vi "Display Dialog.vi"(8 "error in (no error)":errorcluster, 9 "Data":variant, 10 "Argument":string, 11 "State Data":T1) -> (0 "error out":errorcluster, 1 "States at Back":string, 2 "States at Front":string, 3 "State Data out":T1)   [LabVIEW 2020, in "MacroAssert.lvlib"]
doc: "Updates one or more elements of <B>State Data</B> based on <B>Argument</B> and <B>Data</B>."
uses:
  MacroAssert.lvlib
  Classes/Macro/Macro.lvclass
  Custom Errors/Custom Errors.lvlib
  CTLs/Edit Action.ctl
  <vilib>/Utility/miscctls.llb/LVRowAndColumnUnsignedTypeDef.ctl
  <vilib>/Platform/browser.llb/Open URL in Default Browser (string).vi
  CTLs/FGV Actions.ctl
  CTLs/Refs.ctl
  CTLs/Report Data.ctl
  CTLs/Config.ctl
  CTLs/State Data.ctl
  CTLs/App Instance.ctl
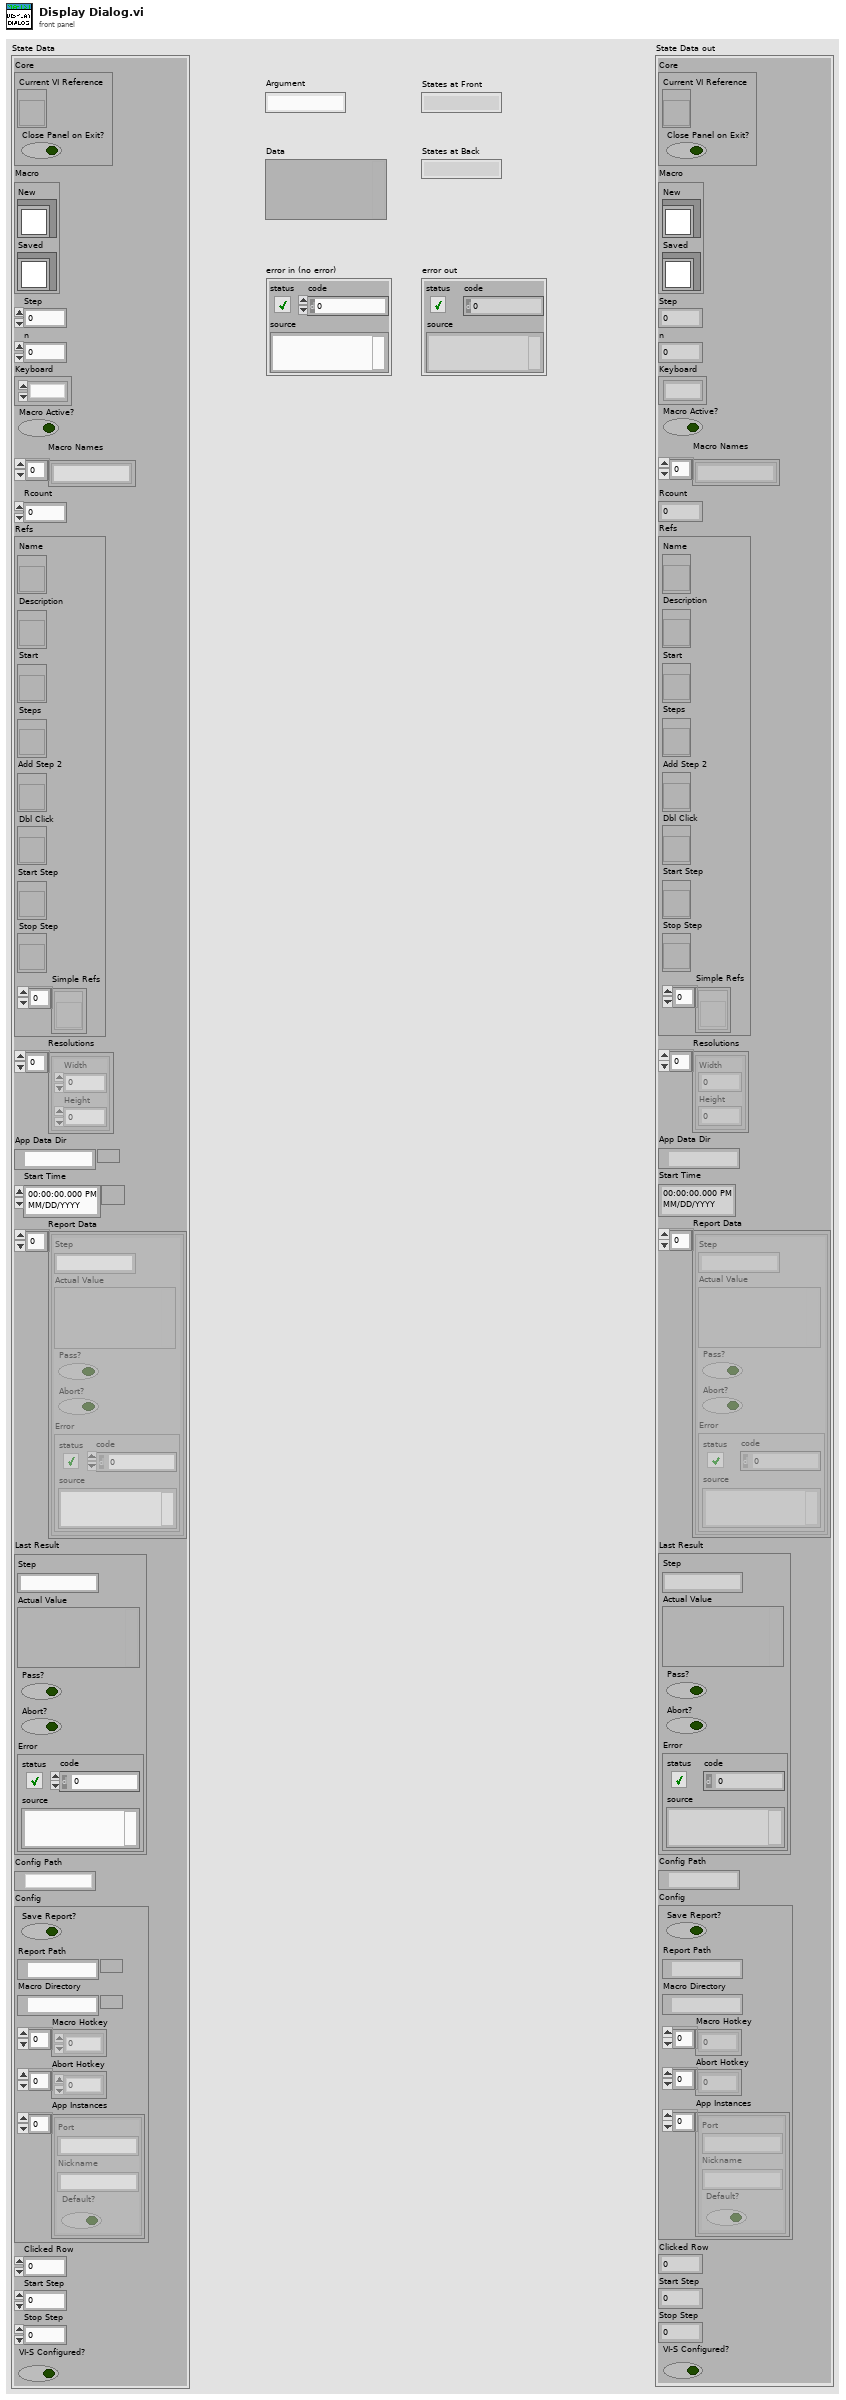
[diagram p1: front panel]
types:
  T1 = typedef "MacroAssert.lvlib/State Data.ctl" = cluster{"Core":cluster{"Current VI Reference":refnum<vi>, "Close Panel on Exit?":bool}, "Macro":cluster{"New":refnum<class "Macro.lvclass">, "Saved":refnum<class "Macro.lvclass">}, "Step":i32, "n":i32, "Keyboard":refnum<k1>, "Macro Active?":bool, "Macro Names":string[], "Rcount":i32, "Refs":T2, "Resolutions":cluster{"Width":i16, "Height":i16}[], "App Data Dir":path, "Start Time":timestamp, "Report Data":T3[], "Last Result":T3, "Config Path":path, "Config":T4, "Clicked Row":i32, "Start Step":i32, "Stop Step":i32, "VI-S Configured?":bool}
  T2 = typedef "MacroAssert.lvlib/Refs.ctl" = cluster{"Name":refnum<vi>, "Description":refnum<vi>, "Start":refnum<vi>, "Steps":refnum<vi>, "Add Step 2":refnum<vi>, "Dbl Click":refnum<vi>, "Start Step":refnum<vi>, "Stop Step":refnum<vi>, "Simple Refs":refnum<vi>[]}
  T3 = typedef "MacroAssert.lvlib/Report Data.ctl" = cluster{"Step":string, "Actual Value":variant, "Pass?":bool, "Abort?":bool, "Error":errorcluster}
  T4 = typedef "MacroAssert.lvlib/Config.ctl" = cluster{"Save Report?":bool, "Report Path":path, "Macro Directory":path, "Macro Hotkey":enum16{"0", "1", "2", "3", "4", "5", "6", "7", "8", "9", "A", "B", "C", "D", "E", "F", "G", "H", "I", "J", "K", "L", "M", "N", "O", "P", "Q", "R", "S", "T", "U", "V", "W", "X", "Y", "Z", "F1", "F2", "F3", "F4", "F5", "F6", "F7", "F8", "F9", "F10", "F11", "F12", "F13", "F14", "F15", "ADD", "BACK", "BACKSLASH", "CAPITAL", "COMMA", "DECIMAL", "DELETE", "DIVIDE", "DOWN", "END", "EQUALS", "ESCAPE", "GRAVE (`)", "HOME", "INSERT", "LBRACKET", "LCONTROL", "LEFT", "L ALT", "LSHIFT", "LWIN", "MINUS", "MULTIPLY", "NEXT", "NUMLOCK", "NUMPAD_0", "NUMPAD_1", "NUMPAD_2", "NUMPAD_3", "NUMPAD_4", "NUMPAD_5", "NUMPAD_6", "NUMPAD_7", "NUMPAD_8", "NUMPAD_9", "PAUSE", "PERIOD", "PRIOR (PG UP)", "RBRACKET", "RCONTROL", "RETURN", "RIGHT", "R ALT", "RSHIFT", "RWIN", "SCROLL", "SEMICOLON", "SLASH", "SPACE", "SUBTRACT", "TAB", "UP", "ENTER (num pad)", "' (quote)"}[], "Abort Hotkey":enum16{"0", "1", "2", "3", "4", "5", "6", "7", "8", "9", "A", "B", "C", "D", "E", "F", "G", "H", "I", "J", "K", "L", "M", "N", "O", "P", "Q", "R", "S", "T", "U", "V", "W", "X", "Y", "Z", "F1", "F2", "F3", "F4", "F5", "F6", "F7", "F8", "F9", "F10", "F11", "F12", "F13", "F14", "F15", "ADD", "BACK", "BACKSLASH", "CAPITAL", "COMMA", "DECIMAL", "DELETE", "DIVIDE", "DOWN", "END", "EQUALS", "ESCAPE", "GRAVE (`)", "HOME", "INSERT", "LBRACKET", "LCONTROL", "LEFT", "L ALT", "LSHIFT", "LWIN", "MINUS", "MULTIPLY", "NEXT", "NUMLOCK", "NUMPAD_0", "NUMPAD_1", "NUMPAD_2", "NUMPAD_3", "NUMPAD_4", "NUMPAD_5", "NUMPAD_6", "NUMPAD_7", "NUMPAD_8", "NUMPAD_9", "PAUSE", "PERIOD", "PRIOR (PG UP)", "RBRACKET", "RCONTROL", "RETURN", "RIGHT", "R ALT", "RSHIFT", "RWIN", "SCROLL", "SEMICOLON", "SLASH", "SPACE", "SUBTRACT", "TAB", "UP", "ENTER (num pad)", "' (quote)"}[], "App Instances":T5[]}
  T5 = typedef "MacroAssert.lvlib/App Instance.ctl" = cluster{"Port":string, "Nickname":string, "Default?":bool}
  T6 = typedef "MacroAssert.lvlib/FGV Actions.ctl" = enum16{"Read", "Write"}
  T7 = typedef "MacroAssert.lvlib/Edit Action.ctl" = enum16{"Add", "Insert", "Modify", "Delete", "Insert Before", "Insert After", "Modify 2", "Delete 2", "Clear All"}
  T8 = typedef "LVRowAndColumnUnsignedTypeDef.ctl" = cluster{"Row":u32, "Column":u32}
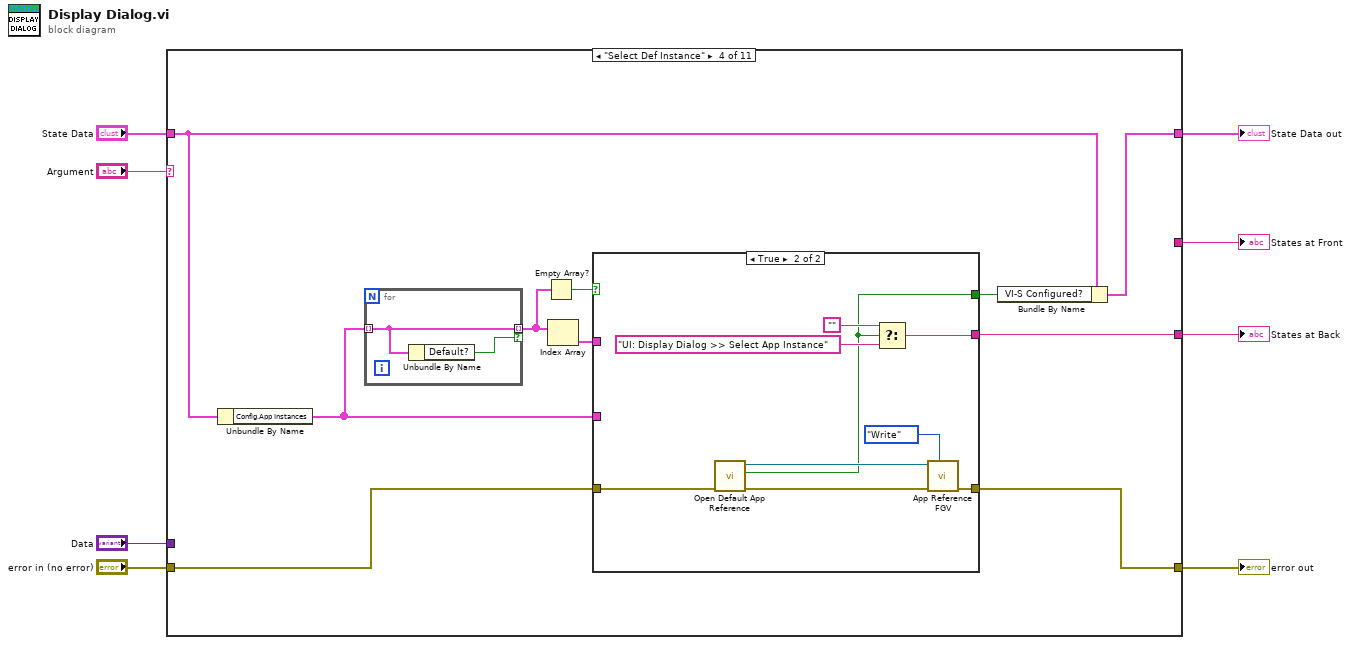
[diagram p0: block diagram]
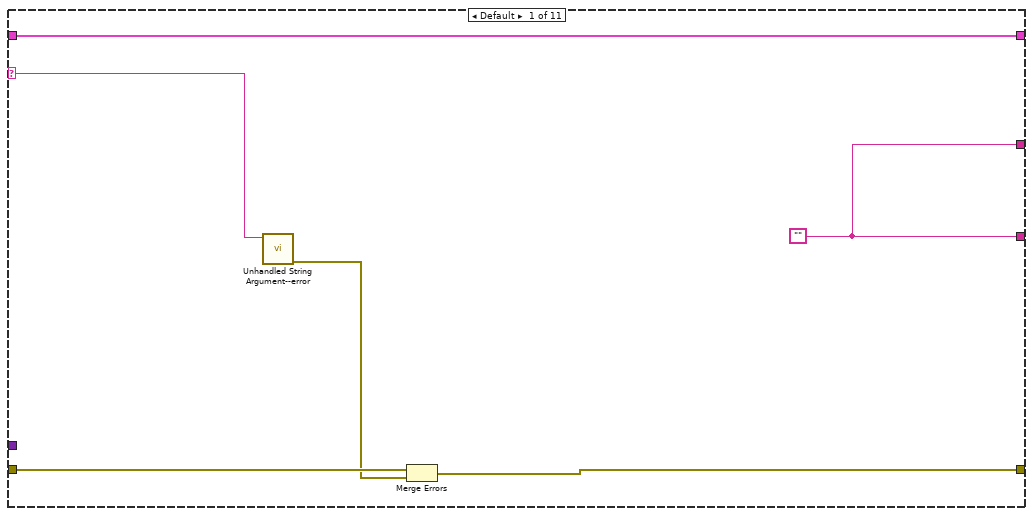
[diagram p2: hidden frame]
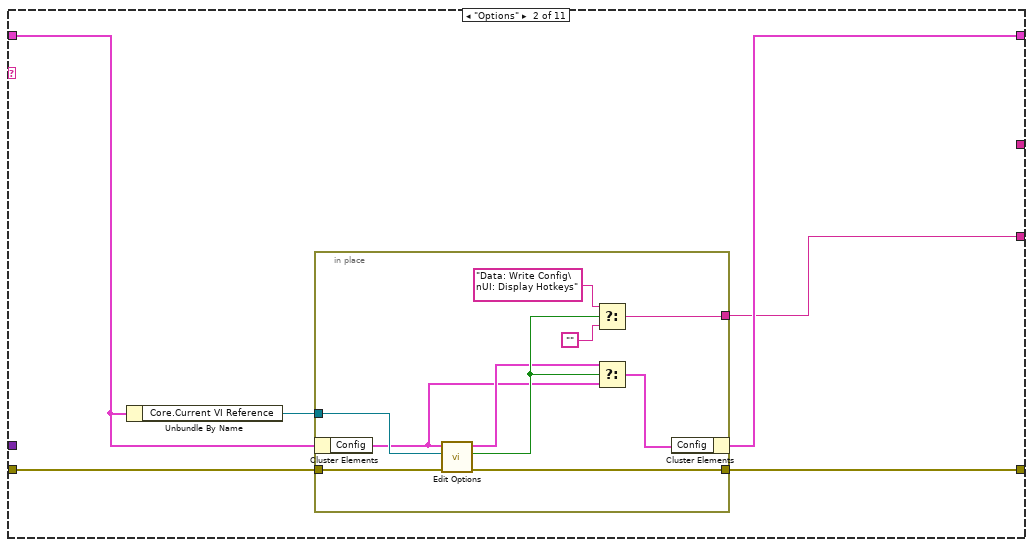
[diagram p3: hidden frame]
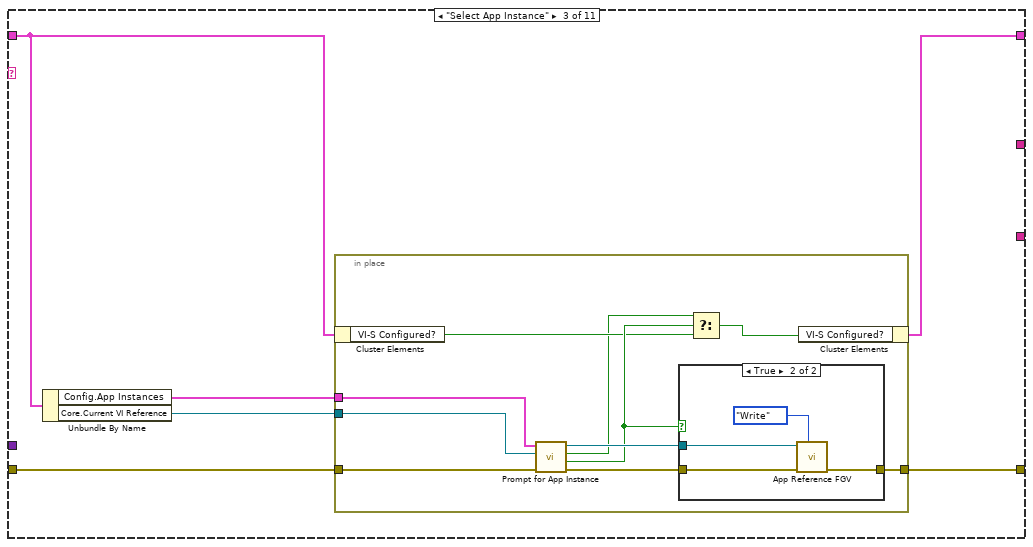
[diagram p4: hidden frame]
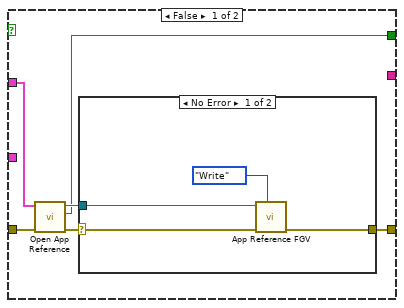
[diagram p6: hidden frame]
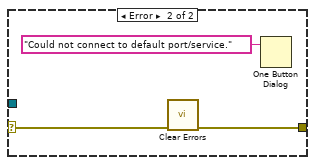
[diagram p7: hidden frame]
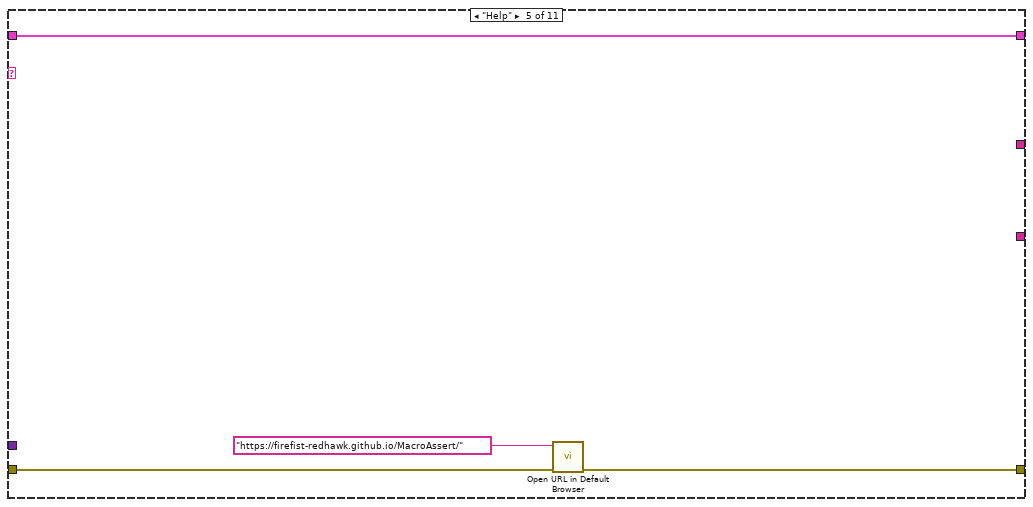
[diagram p8: hidden frame]
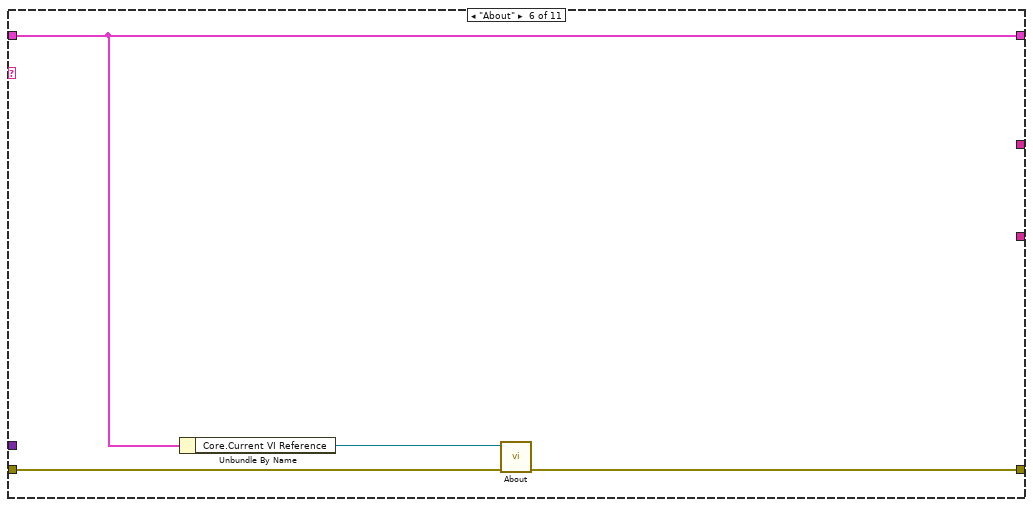
[diagram p9: hidden frame]
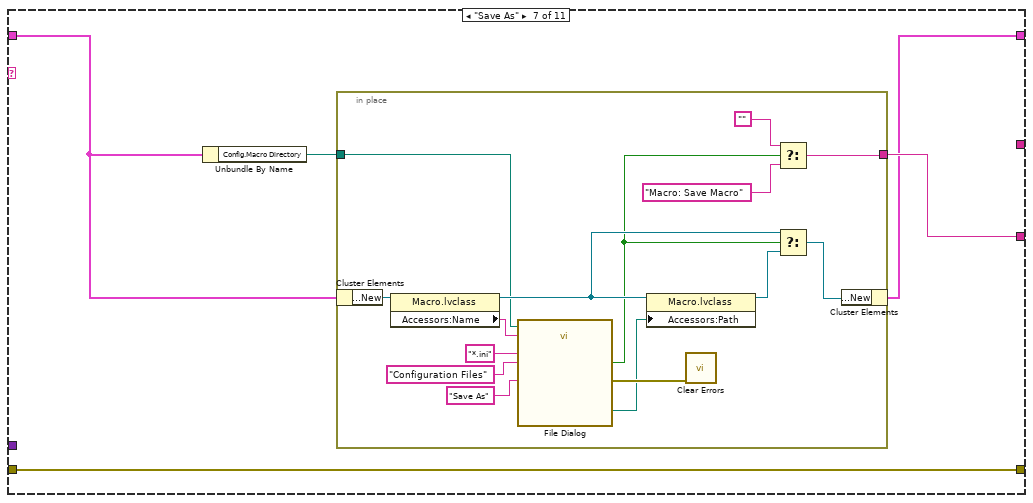
[diagram p10: hidden frame]
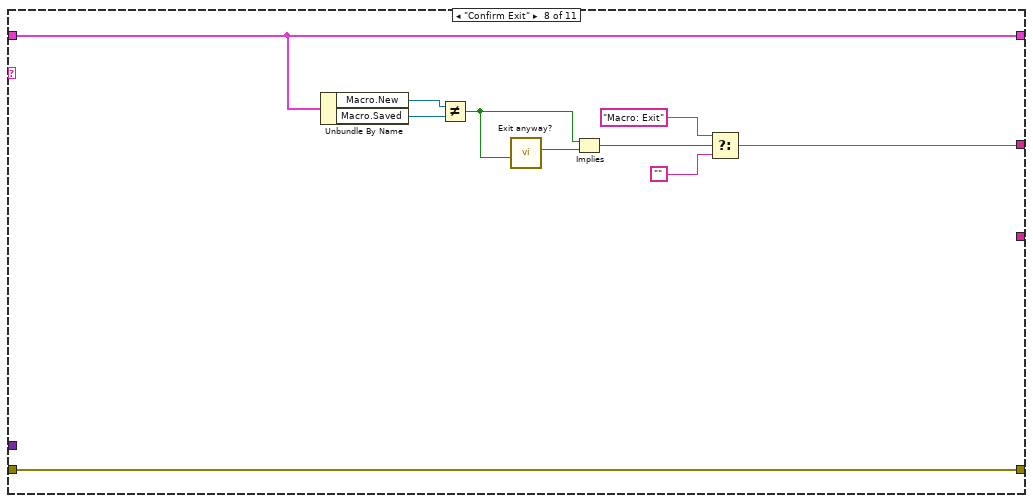
[diagram p11: hidden frame]
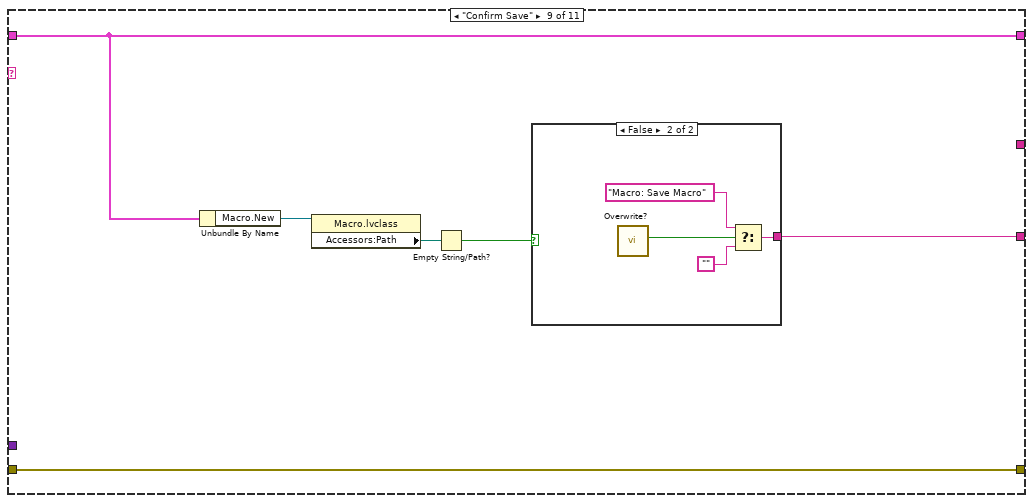
[diagram p12: hidden frame]
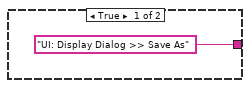
[diagram p13: hidden frame]
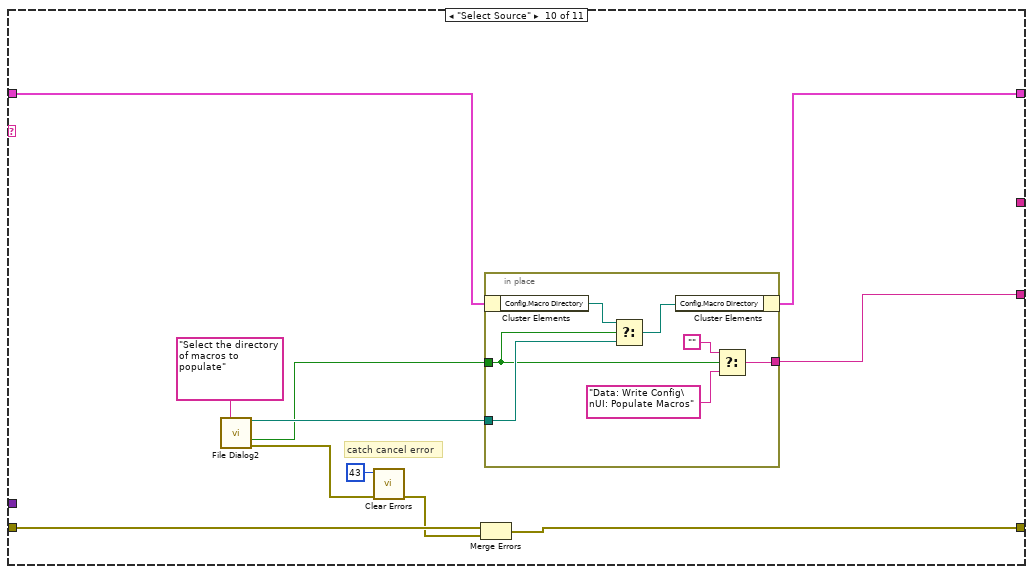
[diagram p14: hidden frame]
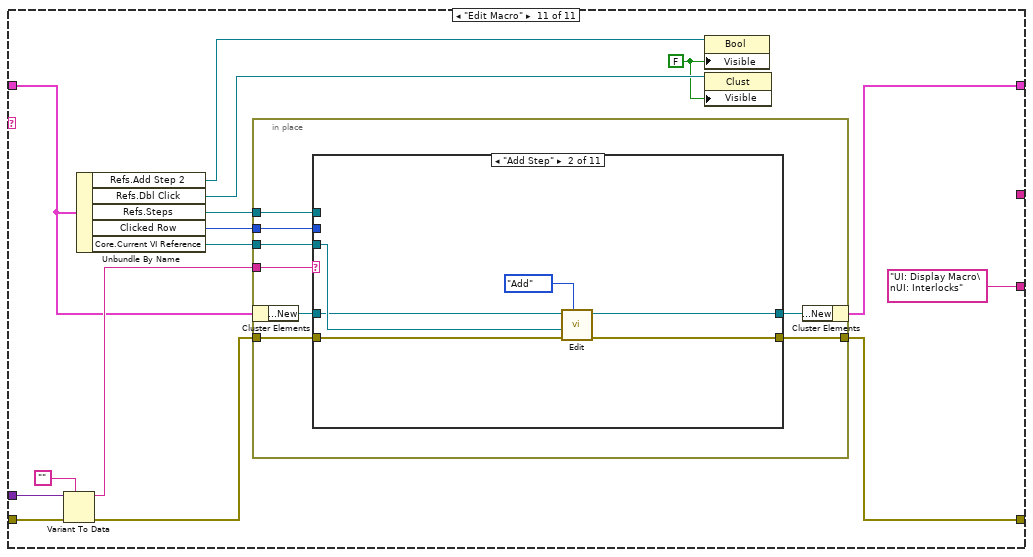
[diagram p15: hidden frame]
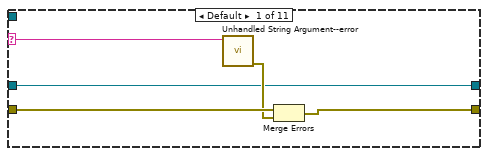
[diagram p16: hidden frame]
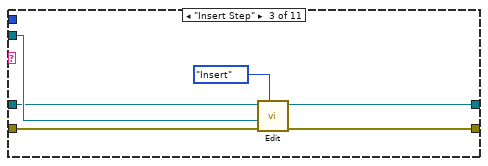
[diagram p17: hidden frame]
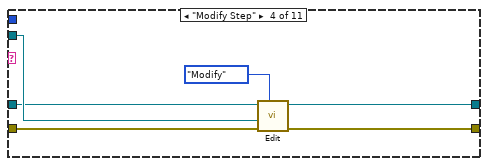
[diagram p18: hidden frame]
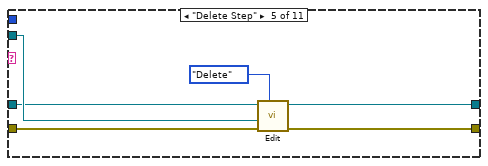
[diagram p19: hidden frame]
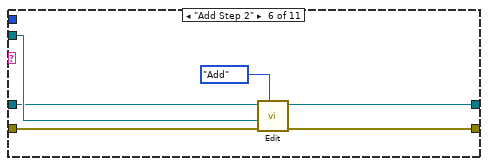
[diagram p20: hidden frame]
diagram:
  n1 = case shown="\"Select Def Instance\"" "Argument" {
    selector: "Argument" -> [w10 _ _ _ _ _ _ _ _ _ _]
    tunnel: "State Data" -> [w11 w15 w32 w54 w89 w91 w96 w118 w125 w138 w155]
    tunnel: "error in (no error)" -> [w14 w20 w36 w61 w87 w93 w98 w123 w129 w144 w167]
    tunnel: "Data" -> [_ _ _ _ _ _ _ _ _ _ w158]
    tunnel: [w11 w17 w31 w52 w89 w91 w94 w118 w125 w137 w159] -> w3
    tunnel: [w9 w16 _ w59 _ _ w95 _ w124 w136 "UI: Display Macro\nUI: Interlocks" ("format string")] -> w2
    tunnel: [w9 _ _ _ _ _ _ w114 _ _ _] -> w1
    tunnel: [w13 w19 w35 w60 w86 w92 w98 w123 w129 w142 w165] -> w7
    frame Default {
      w9 = ""
      n2 = call "Unhandled String Argument--error.vi"("Argument"=w10) -> ("error out"=w12:errorcluster)  [unwired: 10 in]
      n3 = Merge Errors(w14, w12) -> (w13:errorcluster)
    }
    frame "Options" {
      n4 = Unbundle By Name(w15) -> ("Core.Current VI Reference"=w18:refnum<vi>)
      n5 = in-place {
        in-place-border: w20 -> [w30]
        in-place-border: [w29] -> w19
        in-place-border: [w21] -> w16
        in-place-border: w18 -> [w28]
        n6 = in-place-cluster #1(w15) -> ("Config"=w23:T4)
        n7 = call "Edit Options.vi"("error in (no error)"=w30, "Calling VI in"=w28, "Config"=w23) -> ("error out"=w29:errorcluster, "OK?"=w25:bool, "Config out"=w24:T4)  [unwired: 6 in]
        n8 = Select(t="Data: Write Config\nUI: Display Hotkeys", s=w25, f="" ("Empty String Constant")) -> (s? t:f=w21:string)
        n9 = Select(t=w24, s=w25, f=w23) -> (s? t:f=w22:T4)
        n10 = in-place-cluster #1("Config"=w22) -> (w17:T1)
      }
    }
    frame "Select App Instance" {
      n11 = Unbundle By Name(w32) -> ("Config.App Instances"=w33:T5[], "Core.Current VI Reference"=w34:refnum<vi>)
      n12 = in-place {
        in-place-border: w36 -> [w46]
        in-place-border: [w41] -> w35
        in-place-border: w34 -> [w45]
        in-place-border: w33 -> [w44]
        n13 = in-place-cluster #2(w32) -> ("VI-S Configured?"=w39:bool)
        n14 = call "Prompt for App Instance.vi"("error in (no error)"=w46, "Calling VI in"=w45, "App Instances"=w44) -> ("error out"=w43:errorcluster, "OK?"=w40:bool, "VI Server Configured?"=w37:bool, "App Ref"=w42:refnum<vi>)  [unwired: 5 in]
        n15 = case shown="True" w40 {
          tunnel: w43 -> [w47 w50]
          tunnel: w42 -> [_ w49]
          tunnel: [w47 w48] -> w41
          frame False {
          }
          frame True {
            n16 = call "App Reference FGV.vi"("Mode"=FGV_Actions."Write", "error in (no error)"=w50, "App Ref"=w49) -> ("error out"=w48:errorcluster)  [unwired: 7 in, 1 out]
          }
        }
        n17 = Select(t=w37, s=w40, f=w39) -> (s? t:f=w38:bool)
        n18 = in-place-cluster #2("VI-S Configured?"=w38) -> (w31:T1)
      }
    }
    frame "Select Def Instance" {
      n19 = Unbundle By Name(w54) -> ("Config.App Instances"=w57:T5[])
      n20 = for {
        tunnel: w57 -> [w63] mode=indexing
        tunnel: [w63] -> w58 mode=indexing if=w62
        n21 = Unbundle By Name(w63) -> ("Default?"=w62:bool)
      }
      n22 = Empty Array?(array=w58) -> (empty?=w56:bool)
      n23 = Index Array(array=w58) -> (element=w55:T5)  [unwired: 1 in]
      n24 = case shown="True" w56 {
        tunnel: w61 -> [w67 w85]
        tunnel: [w66 w83] -> w60
        tunnel: [_ w78] -> w59
        tunnel: w57 -> [_ _]
        tunnel: w55 -> [w65 _]
        tunnel: [w64 w77] -> w53
        frame False {
          n25 = call "Open App Reference.vi"("error in (no error)"=w67, "App Instance"=w65) -> ("error out"=w68:errorcluster, "VI Server Configured?"=w64:bool, "App Ref"=w69:refnum<vi>)  [unwired: 7 in]
          n26 = case shown="No Error" w68 {
            selector: w68 -> [w72 w76]
            tunnel: w69 -> [w73 _]
            tunnel: [w70 w75] -> w66
            frame No Error {
              n27 = call "App Reference FGV.vi"("Mode"=FGV_Actions."Write", "error in (no error)"=w72, "App Ref"=w73) -> ("error out"=w70:errorcluster)  [unwired: 7 in, 1 out]
            }
            frame Error {
              n28 = call <vilib>:"Clear Errors.vi"("error in (no error)"=w76) -> ("error out"=w75:errorcluster)  [unwired: 5 in, 1 out]
              n29 = One Button Dialog(message="Could not connect to default port/service.") -> ()  [unwired: 1 in, 1 out]
            }
          }
        }
        frame True {
          n30 = call "Open Default App Reference.vi"("error in (no error)"=w85) -> ("error out"=w84:errorcluster, "VI Server Configured?"=w77:bool, "App Ref"=w82:refnum<vi>)  [unwired: 8 in]
          n31 = Select(t="", s=w77, f="UI: Display Dialog >> Select App Instance") -> (s? t:f=w78:string)
          n32 = call "App Reference FGV.vi"("Mode"=FGV_Actions."Write", "error in (no error)"=w84, "App Ref"=w82) -> ("error out"=w83:errorcluster)  [unwired: 7 in, 1 out]
        }
      }
      n33 = Bundle By Name(cluster=w54, "VI-S Configured?"=w53) -> (w52:T1)
    }
    frame "Help" {
      n34 = call-poly <vilib>:"Open URL in Default Browser.vi"("error in (no error)"=w87, "URL"="https://firefist-redhawk.github.io/MacroAssert/") -> ("error out"=w86:errorcluster)  [unwired: 4 in, 1 out]
    }
    frame "About" {
      n35 = Unbundle By Name(w91) -> ("Core.Current VI Reference"=w90:refnum<vi>)
      n36 = call "About.vi"("error in (no error)"=w93, "Calling VI in"=w90) -> ("error out"=w92:errorcluster)  [unwired: 9 in]
    }
    frame "Save As" {
      n37 = Unbundle By Name(w96) -> ("Config.Macro Directory"=w97:path)
      n38 = in-place {
        in-place-border: [w100] -> w95
        in-place-border: w97 -> [w99]
        n39 = in-place-cluster #3(w96) -> ("Macro.New"=w108:refnum<class "Macro.lvclass">)
        n40 = property class="Macro.lvclass"(reference=w108) -> (reference out=w105:refnum<class "Macro.lvclass">, "Accessors:Name"=w109:string)  [unwired: 1 in, 1 out]
        n41 = call "File Dialog"("start path"=w99, "prompt"="Save As", "default name"=w109, "pattern (all files)"="*.ini", "pattern label"="Configuration Files") -> ("selected path"=w107:path, "cancelled"=w103:bool, "error out"=w113:errorcluster)  [unwired: 7 in, 1 out]
        n42 = property class="Macro.lvclass"(reference=w105, "Accessors:Path"=w107) -> (reference out=w106:refnum<class "Macro.lvclass">)  [unwired: 1 in, 1 out]
        n43 = call <vilib>:"Clear Errors.vi"("error in (no error)"=w113) -> ()  [unwired: 5 in, 2 out]
        n44 = Select(t="", s=w103, f="Macro: Save Macro") -> (s? t:f=w100:string)
        n45 = Select(t=w105, s=w103, f=w106) -> (s? t:f=w104:refnum<class "Macro.lvclass">)
        n46 = in-place-cluster #3("Macro.New"=w104) -> (w94:T1)
      }
    }
    frame "Confirm Exit" {
      n47 = Unbundle By Name(w118) -> ("Macro.New"=w120:refnum<class "Macro.lvclass">, "Macro.Saved"=w121:refnum<class "Macro.lvclass">)
      n48 = Not Equal?(x=w120, y=w121) -> (x != y?=w119:bool)
      n49 = call "Exit anyway?"("Enable"=w119) -> ("Exit"=w122:bool)  [unwired: 9 in, 1 out]
      n50 = Implies(1:w122, 2:w119) -> (0:w115:bool)
      n51 = Select(t="Macro: Exit", s=w115, f="") -> (s? t:f=w114:string)
    }
    frame "Confirm Save" {
      n52 = Unbundle By Name(w125) -> ("Macro.New"=w128:refnum<class "Macro.lvclass">)
      n53 = property class="Macro.lvclass"(reference=w128) -> ("Accessors:Path"=w127:path)  [unwired: 1 in, 2 out]
      n54 = Empty String/Path?(string/path=w127) -> (empty?=w126:bool)
      n55 = case shown="False" w126 {
        tunnel: ["UI: Display Dialog >> Save As" w132] -> w124
        frame True {
        }
        frame False {
          n56 = call "Overwrite?"() -> ("OK"=w131:bool)  [unwired: 10 in, 1 out]
          n57 = Select(t="Macro: Save Macro", s=w131, f="") -> (s? t:f=w132:string)
        }
      }
    }
    frame "Select Source" {
      # "catch cancel error"
      n58 = call "File Dialog2"("prompt"="Select the directory of macros to populate") -> ("selected path"=w140:path, "cancelled"=w139:bool, "error out"=w145:errorcluster)  [unwired: 11 in, 1 out]
      n59 = call <vilib>:"Clear Errors.vi"("error in (no error)"=w145, "specific error code to clear (0: all)"=43) -> ("error out"=w143:errorcluster)  [unwired: 4 in, 1 out]
      n60 = Merge Errors(w144, w143) -> (w142:errorcluster)
      n61 = in-place {
        in-place-border: w140 -> [w152]
        in-place-border: w139 -> [w148]
        in-place-border: [w146] -> w136
        n62 = in-place-cluster #4(w138) -> ("Config.Macro Directory"=w151:path)
        n63 = Select(t=w151, s=w148, f=w152) -> (s? t:f=w150:path)
        n64 = in-place-cluster #4("Config.Macro Directory"=w150) -> (w137:T1)
        n65 = Select(t="", s=w148, f="Data: Write Config\nUI: Populate Macros") -> (s? t:f=w146:string)
      }
    }
    frame "Edit Macro" {
      w153 = FALSE ("Visible")
      n66 = Variant To Data(error in=w167, type="", Variant=w158) -> (data=w156:string, error out=w166:errorcluster)
      n67 = Unbundle By Name(w155) -> ("Refs.Add Step 2"=w163:refnum<vi>, "Refs.Dbl Click"=w162:refnum<vi>, "Refs.Steps"=w164:refnum<vi>, "Clicked Row"=w154:i32, "Core.Current VI Reference"=w161:refnum<vi>)
      n68 = in-place {
        in-place-border: w156 -> [w169]
        in-place-border: w154 -> [w168]
        in-place-border: w164 -> [w173]
        in-place-border: w161 -> [w172]
        in-place-border: w166 -> [w175]
        in-place-border: [w174] -> w165
        n69 = in-place-cluster #5(w155) -> ("Macro.New"=w171:refnum<class "Macro.lvclass">)
        n70 = case shown="\"Add Step\"" w169 {
          selector: w169 -> [w176 _ _ _ _ _ _ _ _ _ _]
          tunnel: w171 -> [w177 w182 w188 w194 w200 w207 w212 w219 w227 w234 w242]
          tunnel: [w177 w181 w187 w193 w199 w206 w211 w218 w226 w233 w241] -> w170
          tunnel: w168 -> [_ _ _ _ _ _ w213 w221 w228 w235 _]
          tunnel: w173 -> [_ _ _ _ _ _ _ _ _ _ w244]
          tunnel: w172 -> [_ w184 w190 w196 w202 w208 w215 w223 w230 w237 w243]
          tunnel: w175 -> [w180 w185 w191 w198 w204 w210 w217 w225 w232 w239 w246]
          tunnel: [w178 w186 w192 w197 w203 w209 w216 w224 w231 w238 w245] -> w174
          frame Default {
            n71 = call "Unhandled String Argument--error.vi"("Argument"=w176) -> ("error out"=w179:errorcluster)  [unwired: 10 in]
            n72 = Merge Errors(w180, w179) -> (w178:errorcluster)
          }
          frame "Add Step" {
            n73 = call-dynamic "Edit.vi"("Action"=Edit_Action."Add", "error in (no error)"=w185, "Calling VI in"=w184, "Macro in"=w182) -> ("error out"=w186:errorcluster, "Macro out"=w181:refnum<class "Macro.lvclass">)  [unwired: 6 in]
          }
          frame "Insert Step" {
            n74 = call-dynamic "Edit.vi"("Action"=Edit_Action."Insert", "error in (no error)"=w191, "Calling VI in"=w190, "Macro in"=w188) -> ("error out"=w192:errorcluster, "Macro out"=w187:refnum<class "Macro.lvclass">)  [unwired: 6 in]
          }
          frame "Modify Step" {
            n75 = call-dynamic "Edit.vi"("Action"=Edit_Action."Modify", "error in (no error)"=w198, "Calling VI in"=w196, "Macro in"=w194) -> ("error out"=w197:errorcluster, "Macro out"=w193:refnum<class "Macro.lvclass">)  [unwired: 6 in]
          }
          frame "Delete Step" {
            n76 = call-dynamic "Edit.vi"("Action"=Edit_Action."Delete", "error in (no error)"=w204, "Calling VI in"=w202, "Macro in"=w200) -> ("error out"=w203:errorcluster, "Macro out"=w199:refnum<class "Macro.lvclass">)  [unwired: 6 in]
          }
          frame "Add Step 2" {
            n77 = call-dynamic "Edit.vi"("Action"=Edit_Action."Add", "error in (no error)"=w210, "Calling VI in"=w208, "Macro in"=w207) -> ("error out"=w209:errorcluster, "Macro out"=w206:refnum<class "Macro.lvclass">)  [unwired: 6 in]
          }
          frame "Insert Before" {
            n78 = call-dynamic "Edit.vi"("Action"=Edit_Action."Insert Before", "error in (no error)"=w217, "Calling VI in"=w215, "Step"=w213, "Macro in"=w212) -> ("error out"=w216:errorcluster, "Macro out"=w211:refnum<class "Macro.lvclass">)  [unwired: 5 in]
          }
          frame "Insert After" {
            n79 = Increment(x=w221) -> (x+1=w220:i32)
            n80 = call-dynamic "Edit.vi"("Action"=Edit_Action."Insert After", "error in (no error)"=w225, "Calling VI in"=w223, "Step"=w220, "Macro in"=w219) -> ("error out"=w224:errorcluster, "Macro out"=w218:refnum<class "Macro.lvclass">)  [unwired: 5 in]
          }
          frame "Modify Step 2" {
            n81 = call-dynamic "Edit.vi"("Action"=Edit_Action."Modify 2", "error in (no error)"=w232, "Calling VI in"=w230, "Step"=w228, "Macro in"=w227) -> ("error out"=w231:errorcluster, "Macro out"=w226:refnum<class "Macro.lvclass">)  [unwired: 5 in]
          }
          frame "Delete Step 2" {
            n82 = call-dynamic "Edit.vi"("Action"=Edit_Action."Delete 2", "error in (no error)"=w239, "Calling VI in"=w237, "Step"=w235, "Macro in"=w234) -> ("error out"=w238:errorcluster, "Macro out"=w233:refnum<class "Macro.lvclass">)  [unwired: 5 in]
          }
          frame "Clear Steps" {
            n83 = call "Confirm Clear"() -> ("OK"=w240:bool)  [unwired: 10 in, 1 out]
            n84 = case shown="True" w240 {
              tunnel: w242 -> [w247 w251]
              tunnel: [w247 w250] -> w241
              tunnel: w244 -> [_ w254]
              tunnel: w243 -> [_ w253]
              tunnel: w246 -> [w248 w256]
              tunnel: [w248 w255] -> w245
              frame False {
              }
              frame True {
                n85 = call-dynamic "Edit.vi"("Action"=Edit_Action."Clear All", "error in (no error)"=w256, "Calling VI in"=w253, "Macro in"=w251) -> ("error out"=w255:errorcluster, "Macro out"=w250:refnum<class "Macro.lvclass">)  [unwired: 6 in]
                n86 = property on="Property Node" class="MCListbox"(reference=w254, "TopLeft"=T8 {"Row"=0, "Column"=0} ("Index Values")) -> ()  [unwired: 1 in, 2 out]
              }
            }
          }
        }
        n87 = in-place-cluster #5("Macro.New"=w170) -> (w159:T1)
      }
      n88 = property on="Property Node" class="Bool"(reference=w163, "Visible"=w153) -> ()  [unwired: 1 in, 2 out]
      n89 = property on="Property Node" class="Clust"(reference=w162, "Visible"=w153) -> ()  [unwired: 1 in, 2 out]
    }
  }
  "error out" <- w7
  "State Data out" <- w3
  "States at Back" <- w2
  "States at Front" <- w1
